vi "Tag FGV.vi"(0 "Operation":T4, 5 "Tag Name":string, 9 "Data":variant, 11 "error in (no error)":errorcluster, 12 "Tag Category":string) -> (2 "Alarm Array":T1[](array[typedef]), 3 "Process Name":string, 4 "Tag Names":string[](array[string]), 6 "Tag Values":dbl[](array[numeric]), 10 "Tag Value":dbl, 13 "Boolean alarm settings":T2, 14 "alarms":T3(array[cluster])=[{"alarm URL"="\\\\Nate-VM-LV2018\\sv_alarm_example\\my_number.Alarms.HiHi", "set time"=timestamp(3622821436.098553 s since 1904-01-01), "set user"="(Nobody)", "ack time"=timestamp(-9223372036854775808 s since 1904-01-01), "ack user"="", "clear time"=timestamp(-9223372036854775808 s since 1904-01-01), "clear user"="", "setpoint"=50.0, "value"=97.88238901880113, "priority"=1, "alarm area"="", "alarm description"="", "ack comment"="", "event?"=FALSE, "Refnum"=216172782113783811}] {"value" format="%.2f"; "setpoint" format="%.2f"; "clear time" format="%<%X\n%x>T"; "ack time" format="%<%X\n%x>T"; "set time" format="%<%X\n%x>T"}, 15 "error out":errorcluster)   [LabVIEW 2018, in "Dynamic Shared Variables.lvlib"]
doc: "Handles dynamic tag (shared variable) creation and release as well as alarm configuration and ack."
uses:
  Shared Variables/Dynamic Shared Variables.lvlib
  Tag FGV Operation Enum.ctl
  Numeric Alarm Settings Cluster.ctl
  Utilities/ISO 8601 type.ctl
  Shared Variables/URL Type Enum.ctl
  <vilib>/lvdsc/alarm/Acknowledge Alarms By Instance.vi
  <vilib>/lvdsc/variables/internal/Configure Alarming (Shared Variable, Numeric).vi
  <vilib>/lvdsc/variables/internal/Configure Alarming (Shared Variable, Boolean).vi
  <vilib>/lvdsc/variables/internal/Configure Alarming (Shared Variable, Enable Alarming).vi
  XML Config/XML Config.lvlib
  <vilib>/lvdsc/NI_DSC.lvlib
  <resource>/objmgr/nvio.rc
panel:
  out "Tag Category":string[](array[string])
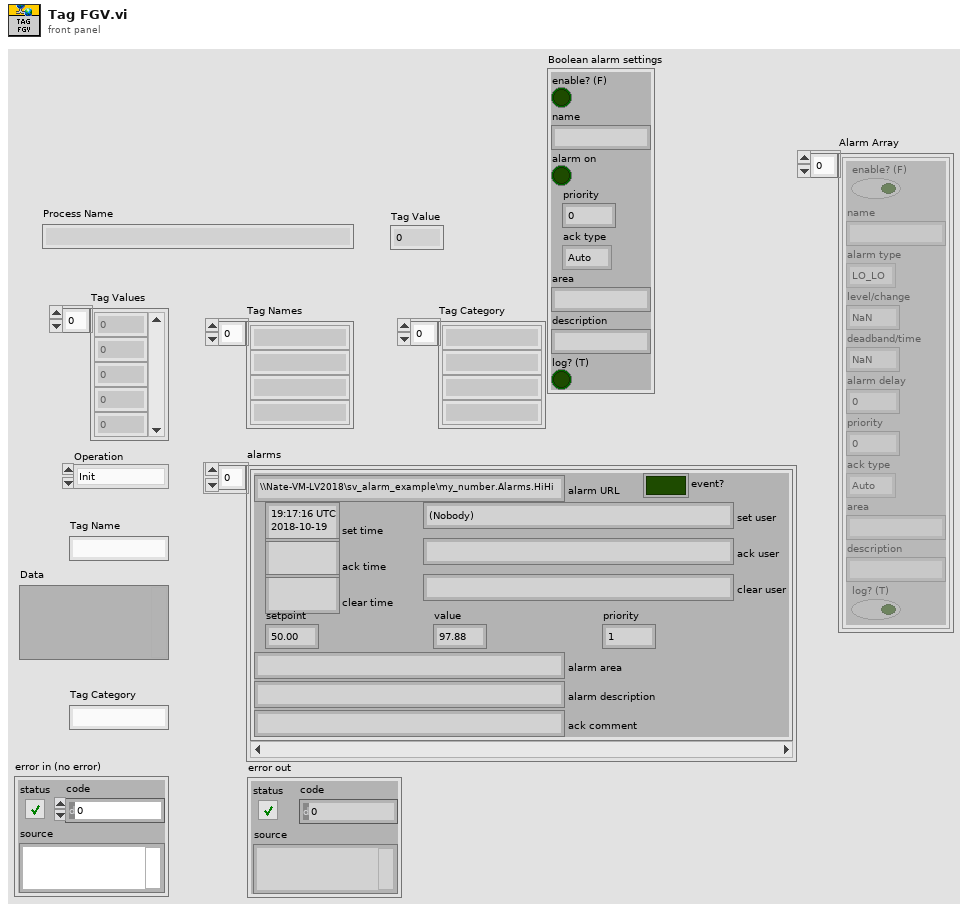
[diagram p1: front panel]
types:
  T1 = typedef "Numeric Alarm Settings Cluster.ctl" = cluster{"enable? (F)":bool, "name":string, "alarm type":enum16{"HI_HI", "HI", "LO", "LO_LO"}, "level/change":dbl, "deadband/time":dbl, "alarm delay":dbl, "priority":u32, "ack type":enum16{"Auto", "User", "None", "Each Occurrence"}, "area":string, "description":string, "log? (T)":bool}
  T2 = cluster{"enable? (F)":bool, "name":string, "alarm on":bool, "priority":u32, "ack type":enum16{"Auto", "User", "None", "Each Occurrence"}, "area":string, "description":string, "log? (T)":bool}
  T3 = cluster{"alarm URL":string, "set time":timestamp, "set user":string, "ack time":timestamp, "ack user":string, "clear time":timestamp, "clear user":string, "setpoint":dbl, "value":dbl, "priority":u32, "alarm area":string, "alarm description":string, "ack comment":string, "event?":bool, "Refnum":u64}[]
  T4 = typedef "Tag FGV Operation Enum.ctl" = enum16{"Init", "Set Notification Queue", "Create Tag", "Commit", "Write Tag (Numeric)", "Write Tag (Boolean)", "Read All Tags", "Read One Tag", "Delete Tag Category", "Set Alarm Parameters (Numeric)", "Set Alarm Parameters (Boolean)", "Enable All Alarms", "Disable All Alarms", "Delete All Tags", "Read Alarms", "Ack Alarm", "Read Alarm Parameters (Numeric)", "Read Alarm Parameters (Boolean)"}
  T5 = typedef "ISO 8601 type.ctl" = enum16{"full ISO 8601 UTC", "basic ISO8601 local", "Windows ISO 8601 UTC", "YYYY-MM-DD UTC", "full ISO 8601 local"}
  T6 = enum32{"u32BitField", "bool", "double", "string", "int8", "uint8", "int16", "uint16", "int32", "uint32", "int64", "uint64", "single", "double waveform", "int16 waveform", "array of boolean", "array of int8", "array of uint8", "array of int16", "array of uint16", "array of int32", "array of uint32", "array of int64", "array of uint64", "array of single", "array of double", "array of double waveform", "array of int16 waveform", "array of string", "variant", "timestamp", "fixed point", "custom"}
  T7 = typedef "Dynamic Shared Variables.lvlib/URL Type Enum.ctl" = enum16{"Tag", "HiHi", "Hi", "Lo", "LoLo", "Tag (Bool)"}
  T8 = cluster{"alarm URL":string, "set time":timestamp, "set user":string, "ack time":timestamp, "ack user":string, "clear time":timestamp, "clear user":string, "setpoint":dbl, "value":dbl, "priority":u32, "alarm area":string, "alarm description":string, "ack comment":string, "event?":bool, "Refnum":u64}
  T9 = enum16{"Auto", "User", "None", "Each Occurrence"}
  T10 = cluster{"enable? (F)":bool, "name":string, "alarm type":enum16{"HI_HI", "HI", "LO", "LO_LO"}, "level/change":dbl, "deadband/time":dbl, "priority":u32, "ack type":enum16{"Auto", "User", "None", "Each Occurrence"}, "area":string, "description":string, "log? (T)":bool}
  T11 = cluster{"enable? (F)":bool, "name":string, "alarm on":bool, "priority":u32, "ack type":enum16{"Auto", "User", "None", "Each Occurrence"}, "area":string, "description":string, "log? (T)":bool}[]
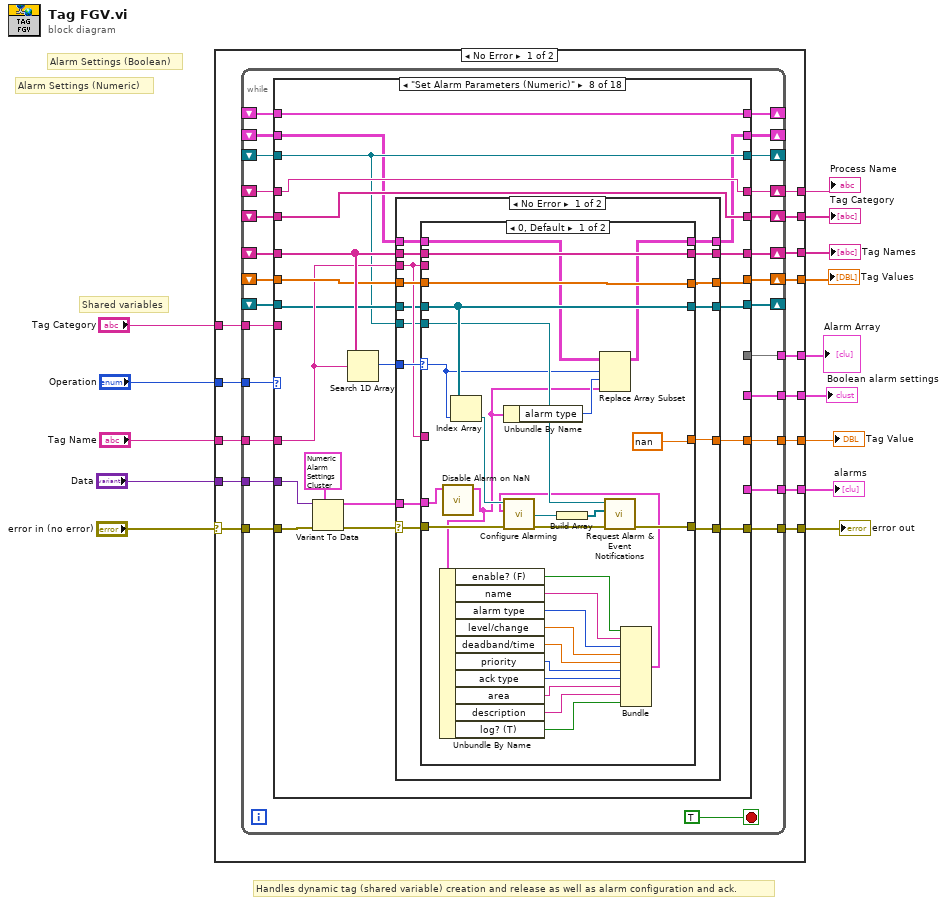
[diagram p0: block diagram]
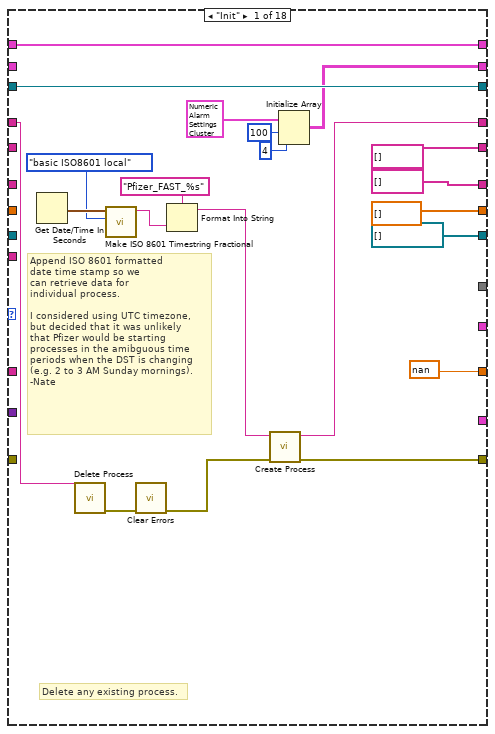
[diagram p2: hidden frame]
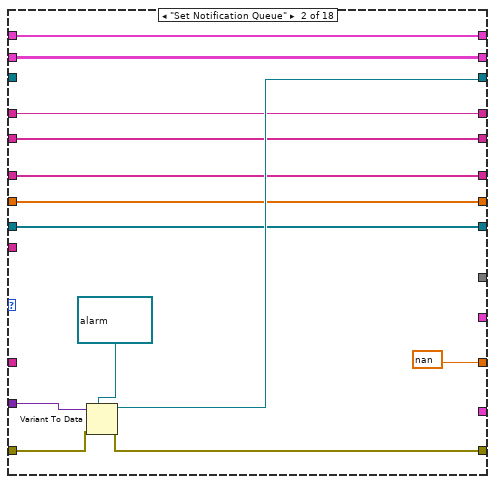
[diagram p3: hidden frame]
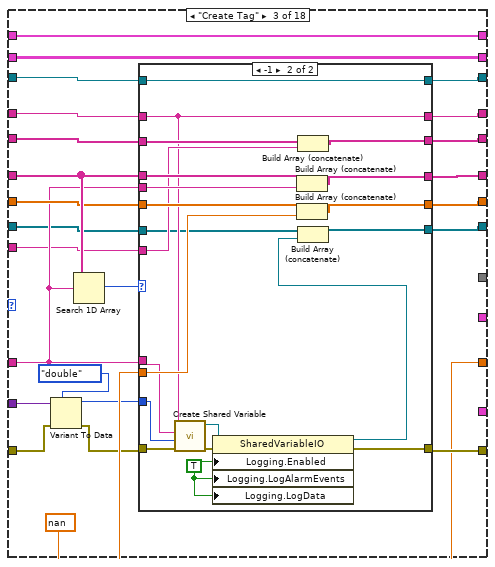
[diagram p4: hidden frame]
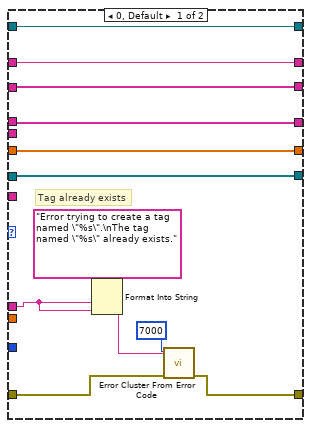
[diagram p5: hidden frame]
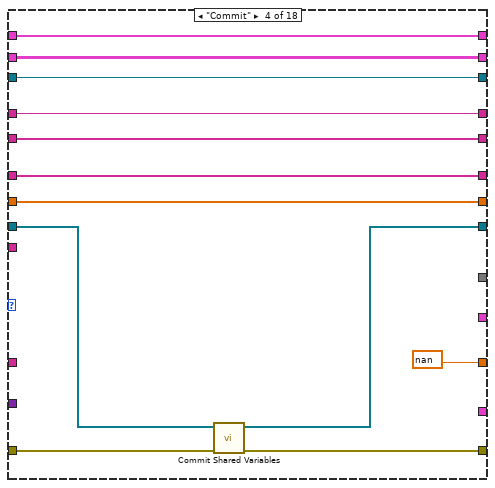
[diagram p6: hidden frame]
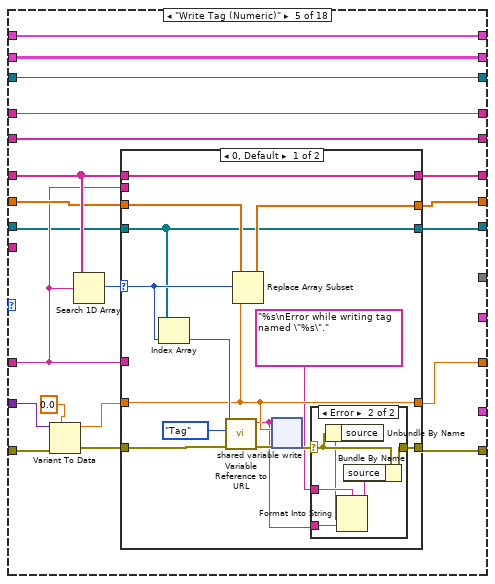
[diagram p7: hidden frame]
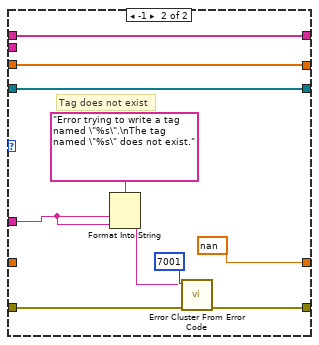
[diagram p9: hidden frame]
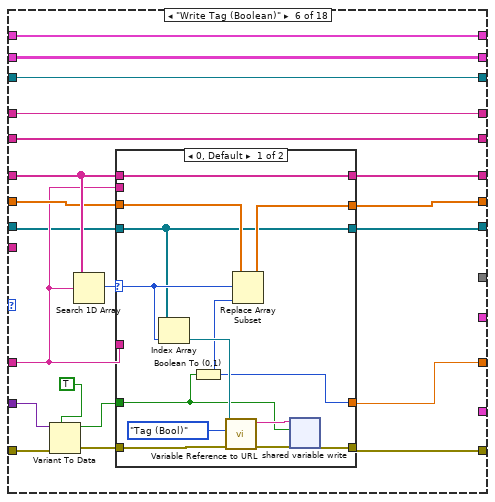
[diagram p10: hidden frame]
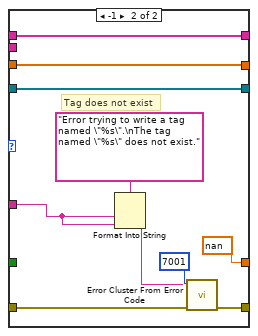
[diagram p11: hidden frame]
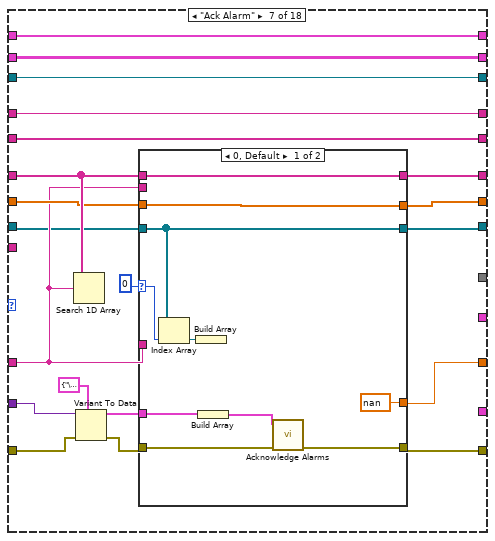
[diagram p12: hidden frame]
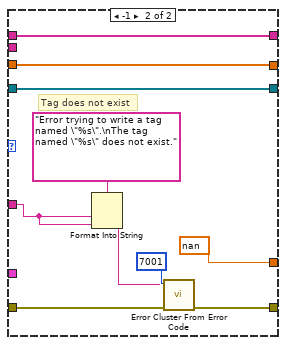
[diagram p13: hidden frame]
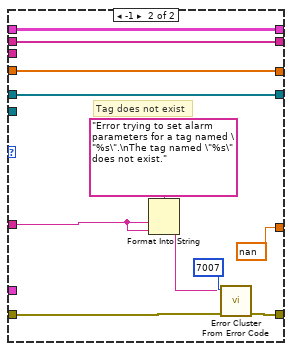
[diagram p14: hidden frame]
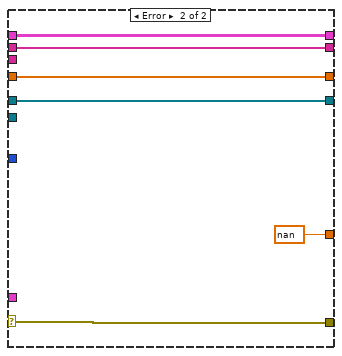
[diagram p15: hidden frame]
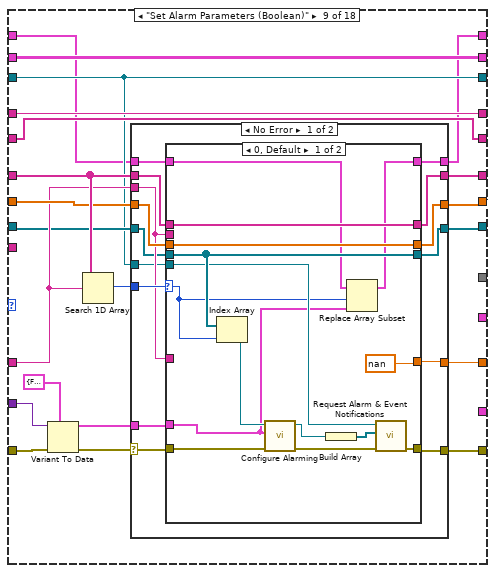
[diagram p16: hidden frame]
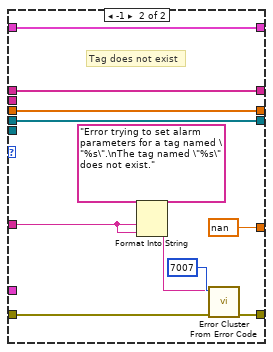
[diagram p17: hidden frame]
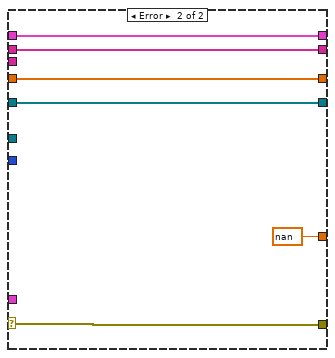
[diagram p18: hidden frame]
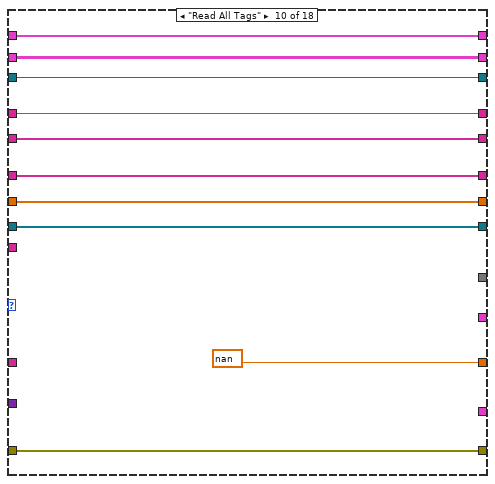
[diagram p19: hidden frame]
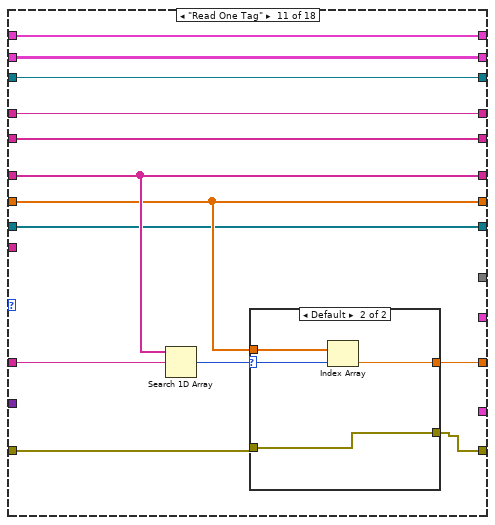
[diagram p20: hidden frame]
diagram:
  # "Alarm Settings (Boolean)"
  # "Alarm Settings (Numeric)"
  # "Handles dynamic tag (shared variable) creation and release as well as alarm configuration and ack."
  # "Shared variables"
  n1 = case shown="No Error" "error in (no error)" {
    selector: "error in (no error)" -> [w25 w618]
    tunnel: [w24 w618] -> w13
    tunnel: "Operation" -> [w28 _]
    tunnel: "Tag Name" -> [w27 _]
    tunnel: "Data" -> [w26 _]
    tunnel: [w23 _] -> w9
    tunnel: [w22 _] -> w8
    tunnel: [w21 nan ("Tag Value (NaN)")] -> w7
    tunnel: "Tag Category" -> [w20 _]
    tunnel: [w19 _] -> w5
    tunnel: [w18 _] -> w4
    tunnel: [w17 _] -> w3
    tunnel: [w16 _] -> w2
    tunnel: [w15 _] -> w1
    frame No Error {
      n2 = while {
        tunnel: w28 -> [w54]
        shift-right: [w52] -> w22
        shift-left: _ -> [w51]
        shift-right: [w53] -> w23
        shift-left: _ -> [w49]
        tunnel: w27 -> [w50]
        tunnel: w26 -> [w48]
        tunnel: w25 -> [w47]
        tunnel: [w45] -> w24
        tunnel: [w46] -> w21
        shift-right: [w44] -> w19
        shift-left: _ -> [w43]
        tunnel: w20 -> [w42]
        shift-right: [w41] -> w17
        shift-left: _ -> [w40]
        shift-right: [w39] -> _
        shift-left: _ -> [w38]
        tunnel: [w37] -> w18
        shift-right: [w36] -> _
        shift-left: _ -> [w35]
        shift-right: [w34] -> _
        shift-left: _ -> [w33]
        shift-right: [w32] -> _
        shift-left: _ -> [w31]
        tunnel: [w30] -> w16
        tunnel: [w29] -> w15
        stop <- TRUE stop-if-true
        n3 = case shown="\"Set Alarm Parameters (Numeric)\"" w54 {
          tunnel: [dbl[] [] ("Tag Values") w84 w109 w157 w174 w225 w269 w309 w390 w451 w462 w481 w497 w513 dbl[] [] ("Tag Values") w559 w576 w603] -> w53
          tunnel: [string[] [] ("Tag Names") w82 w111 w158 w176 w227 w271 w311 w392 w450 w464 w482 w498 w515 w543 w558 w572 w599] -> w52
          tunnel: w51 -> [_ w82 w112 w158 w177 w228 w272 w312 w393 w450 w464 w482 w498 w516 _ w558 w572 w599]
          tunnel: w50 -> [_ _ w108 _ w173 w224 w268 w308 w389 _ w463 _ _ w520 _ _ w567 w593]
          tunnel: w49 -> [_ w84 w110 w157 w175 w226 w270 w310 w391 w451 w462 w481 w497 w514 _ w559 w576 w603]
          tunnel: w48 -> [_ w88 w98 _ w162 w213 w261 w300 w381 _ _ _ _ _ _ _ _ _]
          tunnel: w47 -> [_ w86 w96 w150 w165 w216 w259 w298 w379 w449 w458 w477 w493 w510 w537 w563 w570 w597]
          tunnel: [w72 w85 w107 w156 w172 w223 w267 w307 w388 w449 w459 w475 w491 w508 w540 w562 w569 w596] -> w45
          tunnel: [nan ("Tag Value (NaN)") nan ("Tag Value (NaN)") w99 nan ("Tag Value (NaN)") w171 w222 w266 w306 w387 nan ("Tag Value (NaN)") w461 nan nan nan ("Tag Value (NaN)") nan ("Tag Value (NaN)") nan ("Tag Value (NaN)") nan ("Tag Value (NaN)") nan ("Tag Value (NaN)")] -> w46
          tunnel: [string[] [] ("Tag Names") w81 w104 w155 w170 w221 w265 w305 w386 w447 w457 w480 w496 w517 w543 w557 w577 w604] -> w44
          tunnel: w43 -> [_ w81 w106 w155 w170 w221 w265 w305 w386 w447 w457 w480 w496 w518 _ w557 w577 w604]
          tunnel: w42 -> [_ _ w105 _ _ _ _ _ _ _ _ _ _ w519 w546 _ _ _]
          tunnel: [w71 w80 w102 w154 w168 w219 w263 w303 w384 w445 w455 w479 w495 w507 w536 w556 w578 w605] -> w41
          tunnel: w40 -> [w62 w80 w103 w154 w168 w219 w263 w303 w384 w445 w455 w479 w495 w507 w536 w556 w578 w605]
          tunnel: [refnum<k21>[] [] w83 w101 w153 w167 w218 w262 w302 w383 w446 w456 w478 w494 w506 refnum<k21>[] [] w560 w575 w602] -> w39
          tunnel: w38 -> [_ w83 w100 w152 w169 w220 w264 w304 w385 w446 w456 w478 w494 w511 w544 w560 w575 w602]
          tunnel: [_ _ _ _ _ _ _ _ _ _ _ _ _ _ _ w564 _ _] -> w37
          tunnel: [w64 w87 w93 w151 w161 w212 w255 w297 w377 w444 w454 w473 w489 w505 w539 w555 w571 w598] -> w36
          tunnel: w35 -> [w64 _ w92 w151 w161 w212 w255 w297 w377 w444 w454 w473 w489 w505 w539 w555 w571 w598]
          tunnel: [w56 w78 w91 w148 w160 w211 w254 w296 w376 w443 w453 w472 w488 w504 w534 w554 w568 w606] -> w34
          tunnel: w33 -> [_ w78 w91 w148 w160 w211 w254 w295 w376 w443 w453 w472 w488 w504 w534 w554 w568 w606]
          tunnel: [w60 w77 w90 w147 w159 w210 w253 w294 w375 w442 w452 w471 w487 w503 w533 w553 w579 w595] -> w32
          tunnel: w31 -> [w60 w77 w90 w147 w159 w210 w253 w294 w374 w442 w452 w471 w487 w503 w533 w553 w579 w595]
          tunnel: [_ _ _ _ _ _ _ _ _ _ _ _ _ _ _ _ _ w594] -> w30
          tunnel: [_ _ _ _ _ _ _ _ _ _ _ _ _ _ _ _ w566 _] -> w29
          frame "Init" {
            # "Delete any existing process."
            # "Append ISO 8601 formatted\ndate time stamp so we\ncan retrieve data for\nindividual process.\n\nI considered using UTC timezone,\nbut decided that it was unlikely\nthat Pfizer would be starting\nprocesses in the amibguous time\nperiods when the DST is changing\n(e.g. 2 to 3 AM Sunday mornings).\n-Nate"
            n4 = Get Date/Time In Seconds() -> (seconds since 1Jan1904=w69:timestamp)
            n5 = call <vilib>:"Delete Process.vi"("process name"=w62) -> ("error out"=w63:errorcluster)  [unwired: 10 in]
            n6 = call "Make ISO 8601 Timestring Fractional.vi"("ISO 8601 type"=ISO_8601_type."basic ISO8601 local", "Time Stamp"=w69) -> ("ISO 8601 Timestring"=w66:string)  [unwired: 8 in, 1 out]
            n7 = call <vilib>:"Clear Errors.vi"("error in (no error)"=w63) -> ("error out"=w61:errorcluster)  [unwired: 5 in, 1 out]
            n8 = Format Into String(format string="Pfizer_FAST_%s", w66) -> (resulting string=w65:string)  [unwired: 2 in, 1 out]
            n9 = call "Create Process.vi"("error in (no error)"=w61, "process name"=w65) -> ("error out"=w72:errorcluster, "dup process name"=w71:string)  [unwired: 8 in]
            n10 = Initialize Array(T1 {"enable? (F)"=FALSE, "name"="", "alarm type"=enum."LO_LO", "level/change"=nan, "deadband/time"=nan, "alarm delay"=0.0, "priority"=0, "ack type"=enum."Auto", "area"="", "description"="", "log? (T)"=FALSE} ("numeric alarm settings out"), 100 ("dimension size"), 4 ("dimension size")) -> (w56:T1[][])
          }
          frame "Set Notification Queue" {
            n11 = Variant To Data(error in=w86, type=refnum<user-event> refnum ("notification refnum"), Variant=w88) -> (data=w87:refnum<user-event>, error out=w85:errorcluster)
          }
          frame "Create Tag" {
            w99 = nan ("Tag Value (NaN)")
            n12 = Variant To Data(error in=w96, type=T6."double" ("data type"), Variant=w98) -> (data=w94:T6, error out=w97:errorcluster)
            n13 = Search 1D Array(1D array=w112, element=w108) -> (index of element=w113:i32)  [unwired: 1 in]
            n14 = case shown="-1" w113 {
              tunnel: w108 -> [_ w146]
              tunnel: w112 -> [w125 w145]
              tunnel: [w125 w144] -> w111
              tunnel: w110 -> [w124 w143]
              tunnel: w99 -> [_ w142]
              tunnel: [w124 w141] -> w109
              tunnel: w97 -> [w123 w136]
              tunnel: w108 -> [w120 w137]
              tunnel: [w118 w126] -> w107
              tunnel: w106 -> [w117 w140]
              tunnel: w105 -> [_ w139]
              tunnel: [w117 w138] -> w104
              tunnel: w103 -> [w116 w135]
              tunnel: [w116 w135] -> w102
              tunnel: [w115 w134] -> w101
              tunnel: w100 -> [w115 w133]
              tunnel: w94 -> [_ w129]
              tunnel: [w114 w127] -> w93
              tunnel: w92 -> [w114 w127]
              frame 0, Default {
                # "Tag already exists"
                n15 = Format Into String(format string="Error trying to create a tag named \"%s\".\nThe tag named \"%s\" already exists.", w120, w120) -> (resulting string=w119:string)  [unwired: 2 in, 1 out]
                n16 = call <vilib>:"Error Cluster From Error Code.vi"("error in (no error)"=w123, "error message (\"\")"=w119, "error code (0)"=7000) -> ("error out"=w118:errorcluster)  [unwired: 6 in]
              }
              frame -1 {
                w130 = TRUE ("Logging.LogAlarmEvents")
                n17 = call "Create Shared Variable.vi"("error in (no error)"=w136, "data type"=w129, "shared variable name"=w137, "process name out"=w135) -> ("error out"=w132:errorcluster, "shared variable"=w128:refnum<k21>)  [unwired: 6 in]
                n18 = property class="SharedVariableIO"(reference=w128, error in=w132, "Logging.Enabled"=w130, "Logging.LogAlarmEvents"=w130, "Logging.LogData"=w130) -> (reference out=w131:refnum<k21>, error out=w126:errorcluster)
                n19 = Build Array (concatenate)(w145, w146) -> (w144:string[])
                n20 = Build Array (concatenate)(w143, w142) -> (w141:dbl[])
                n21 = Build Array (concatenate)(w140, w139) -> (w138:string[])
                n22 = Build Array (concatenate)(w133, w131) -> (w134:refnum<k21>[])
              }
            }
          }
          frame "Commit" {
            n23 = call <vilib>:"Commit Shared Variables.vi"("error in (no error)"=w150, "shared variables"=w152) -> ("error out"=w156:errorcluster, "shared variables out"=w153:refnum<k21>[])  [unwired: 8 in]
          }
          frame "Write Tag (Numeric)" {
            n24 = Variant To Data(error in=w165, type=0.0, Variant=w162) -> (data=w163:dbl, error out=w164:errorcluster)
            n25 = Search 1D Array(1D array=w177, element=w173) -> (index of element=w178:i32)  [unwired: 1 in]
            n26 = case shown="0, Default" w178 {
              selector: w178 -> [w189 _]
              tunnel: w173 -> [_ _]
              tunnel: w177 -> [w192 w209]
              tunnel: [w192 w209] -> w176
              tunnel: w175 -> [w191 w208]
              tunnel: w163 -> [w186 _]
              tunnel: [w190 w208] -> w174
              tunnel: w164 -> [w185 w207]
              tunnel: w173 -> [_ w204]
              tunnel: [w181 w202] -> w172
              tunnel: [w186 nan ("Tag Value (NaN)")] -> w171
              tunnel: w169 -> [w183 w200]
              tunnel: [w183 w200] -> w167
              frame 0, Default {
                n27 = Index Array(array=w183, index=w189) -> (element=w188:refnum<k21>)
                n28 = call "Variable Reference to URL.vi"("error in (no error)"=w185, "URL type"=URL_Type_Enum."Tag", "variable reference"=w188) -> ("error out"=w184:errorcluster, "URL"=w179:string)  [unwired: 7 in]
                n29 = Replace Array Subset(array=w191, new element=w186, index=w189) -> (w190:dbl[])
                n30 = shared-variable-write(w179, w184, w186) -> (w182:errorcluster)  [unwired: 1 out]
                n31 = case shown="Error" w182 {
                  selector: w182 -> [w193 w199]
                  tunnel: [w193 w198] -> w181
                  tunnel: "%s\nError while writing tag named \"%s\"." ("format string") -> [_ w197]
                  tunnel: w179 -> [_ w194]
                  frame No Error {
                  }
                  frame Error {
                    n32 = Unbundle By Name(w199) -> ("source"=w196:string)
                    n33 = Format Into String(format string=w197, w196, w194) -> (resulting string=w195:string)  [unwired: 2 in, 1 out]
                    n34 = Bundle By Name(cluster=w199, "source"=w195) -> (w198:errorcluster)
                  }
                }
              }
              frame -1 {
                # "Tag does not exist"
                n35 = Format Into String(format string="Error trying to write a tag named \"%s\".\nThe tag named \"%s\" does not exist.", w204, w204) -> (resulting string=w203:string)  [unwired: 2 in, 1 out]
                n36 = call <vilib>:"Error Cluster From Error Code.vi"("error in (no error)"=w207, "error message (\"\")"=w203, "error code (0)"=7001) -> ("error out"=w202:errorcluster)  [unwired: 6 in]
              }
            }
          }
          frame "Write Tag (Boolean)" {
            n37 = Variant To Data(error in=w216, type=TRUE, Variant=w213) -> (data=w214:bool, error out=w215:errorcluster)
            n38 = Search 1D Array(1D array=w228, element=w224) -> (index of element=w229:i32)  [unwired: 1 in]
            n39 = case shown="0, Default" w229 {
              selector: w229 -> [w239 _]
              tunnel: w224 -> [_ _]
              tunnel: w228 -> [w242 w252]
              tunnel: [w242 w252] -> w227
              tunnel: w226 -> [w241 w251]
              tunnel: w214 -> [w231 _]
              tunnel: [w240 w251] -> w225
              tunnel: w215 -> [w235 w250]
              tunnel: w224 -> [_ w247]
              tunnel: [w233 w245] -> w223
              tunnel: [w230 nan ("Tag Value (NaN)")] -> w222
              tunnel: w220 -> [w232 w243]
              tunnel: [w232 w243] -> w218
              frame 0, Default {
                n40 = Index Array(array=w232, index=w239) -> (element=w238:refnum<k21>)
                n41 = Boolean To (0,1)(Boolean=w231) -> (0, 1=w230:i16)
                n42 = call "Variable Reference to URL.vi"("error in (no error)"=w235, "URL type"=URL_Type_Enum."Tag (Bool)", "variable reference"=w238) -> ("error out"=w234:errorcluster, "URL"=w236:string)  [unwired: 7 in]
                n43 = Replace Array Subset(array=w241, new element=w230, index=w239) -> (w240:dbl[])
                n44 = shared-variable-write(w236, w234, w231) -> (w233:errorcluster)  [unwired: 1 out]
              }
              frame -1 {
                # "Tag does not exist"
                n45 = Format Into String(format string="Error trying to write a tag named \"%s\".\nThe tag named \"%s\" does not exist.", w247, w247) -> (resulting string=w246:string)  [unwired: 2 in, 1 out]
                n46 = call <vilib>:"Error Cluster From Error Code.vi"("error in (no error)"=w250, "error message (\"\")"=w246, "error code (0)"=7001) -> ("error out"=w245:errorcluster)  [unwired: 6 in]
              }
            }
          }
          frame "Ack Alarm" {
            n47 = Search 1D Array(1D array=w272, element=w268) -> ()  [unwired: 1 in, 1 out]
            n48 = Variant To Data(error in=w259, type=T8 {"alarm URL"="\\\\Nate-VM-LV2018\\Pfizer FAST\\TT1.Alarms.TT1:LoLo", "set time"=timestamp(3634824876.5239263 s since 1904-01-01), "set user"="(Nobody)", "ack time"=timestamp(-9223372036854775808 s since 1904-01-01), "ack user"="", "clear time"=timestamp(-9223372036854775808 s since 1904-01-01), "clear user"="", "setpoint"=20.0, "value"=19.923748781652513, "priority"=100, "alarm area"="", "alarm description"="", "ack comment"="", "event?"=FALSE, "Refnum"=216172782113783885} ("Alarm"), Variant=w261) -> (data=w258:T8, error out=w260:errorcluster)
            n49 = case shown="0, Default" 0 ("index of element") {
              selector: 0 ("index of element") -> [w281 _]
              tunnel: w268 -> [_ _]
              tunnel: w272 -> [w282 w292]
              tunnel: [w282 w292] -> w271
              tunnel: w270 -> [w278 w291]
              tunnel: [w278 w291] -> w269
              tunnel: w260 -> [w276 w290]
              tunnel: w268 -> [_ w287]
              tunnel: [w275 w285] -> w267
              tunnel: [nan ("Tag Value (NaN)") nan ("Tag Value (NaN)")] -> w266
              tunnel: w264 -> [w280 w283]
              tunnel: [w280 w283] -> w262
              tunnel: w258 -> [w274 _]
              frame 0, Default {
                n50 = Index Array(array=w280, index=w281) -> (element=w279:refnum<k21>)
                n51 = Build Array(w279) -> ()  [unwired: 1 out]
                n52 = Build Array(w274) -> (w273:T3)
                n53 = call-poly <vilib>:"Acknowledge Alarms.vi"("error in (no error)"=w276, "alarms"=w273) -> ("error out"=w275:errorcluster)  [unwired: 9 in]
              }
              frame -1 {
                # "Tag does not exist"
                n54 = Format Into String(format string="Error trying to write a tag named \"%s\".\nThe tag named \"%s\" does not exist.", w287, w287) -> (resulting string=w286:string)  [unwired: 2 in, 1 out]
                n55 = call <vilib>:"Error Cluster From Error Code.vi"("error in (no error)"=w290, "error message (\"\")"=w286, "error code (0)"=7001) -> ("error out"=w285:errorcluster)  [unwired: 6 in]
              }
            }
          }
          frame "Set Alarm Parameters (Numeric)" {
            n56 = Variant To Data(error in=w298, type=T1 {"enable? (F)"=FALSE, "name"="", "alarm type"=enum."LO_LO", "level/change"=nan, "deadband/time"=nan, "alarm delay"=0.0, "priority"=0, "ack type"=enum."Auto", "area"="", "description"="", "log? (T)"=FALSE} ("numeric alarm settings out"), Variant=w300) -> (data=w301:T1, error out=w299:errorcluster)
            n57 = Search 1D Array(1D array=w312, element=w308) -> (index of element=w313:i32)  [unwired: 1 in]
            n58 = case shown="No Error" w299 {
              selector: w299 -> [w317 w369]
              tunnel: w313 -> [w328 _]
              tunnel: w312 -> [w327 w371]
              tunnel: [w326 w371] -> w311
              tunnel: w310 -> [w325 w372]
              tunnel: w301 -> [w324 _]
              tunnel: [w323 w372] -> w309
              tunnel: w308 -> [w322 _]
              tunnel: [w321 w369] -> w307
              tunnel: [w320 nan ("Tag Value (NaN)")] -> w306
              tunnel: w304 -> [w319 w373]
              tunnel: [w318 w373] -> w302
              tunnel: w297 -> [w316 _]
              tunnel: [w315 w368] -> w296
              tunnel: w295 -> [w314 w368]
              frame No Error {
                n59 = case shown="0, Default" w328 {
                  selector: w328 -> [w344 _]
                  tunnel: w322 -> [_ _]
                  tunnel: w327 -> [w356 w367]
                  tunnel: [w356 w367] -> w326
                  tunnel: w325 -> [w351 w366]
                  tunnel: w324 -> [w350 _]
                  tunnel: [w351 w366] -> w323
                  tunnel: w317 -> [w353 w365]
                  tunnel: w322 -> [_ w358]
                  tunnel: [w345 w361] -> w321
                  tunnel: [nan nan ("Tag Value (NaN)")] -> w320
                  tunnel: w319 -> [w355 w359]
                  tunnel: [w355 w359] -> w318
                  tunnel: w316 -> [w347 _]
                  tunnel: [w343 w357] -> w315
                  tunnel: w314 -> [w342 w357]
                  frame 0, Default {
                    n60 = call "Disable Alarm on NaN.vi"("numeric alarm settings in"=w350) -> ("numeric alarm settings out"=w340:T1)  [unwired: 10 in]
                    n61 = Unbundle By Name(w340) -> ("enable? (F)"=w339:bool, "name"=w338:string, "alarm type"=w337:enum16{"HI_HI", "HI", "LO", "LO_LO"}, "level/change"=w336:dbl, "deadband/time"=w335:dbl, "priority"=w334:u32, "ack type"=w333:T9, "area"=w332:string, "description"=w331:string, "log? (T)"=w330:bool)
                    n62 = Index Array(array=w355, index=w344) -> (element=w354:refnum<k21>)
                    n63 = Unbundle By Name(w340) -> ("alarm type"=w341:enum16{"HI_HI", "HI", "LO", "LO_LO"})
                    n64 = Replace Array Subset(array=w342, new element=w340, index (row)=w344, index (col)=w341) -> (w343:T1[][])
                    n65 = Bundle("enable? (F)"=w339, "name"=w338, "alarm type"=w337, "level/change"=w336, "deadband/time"=w335, "priority"=w334, "ack type"=w333, "area"=w332, "description"=w331, "log? (T)"=w330) -> (w329:T10)  [unwired: 1 in]
                    n66 = call-poly <vilib>:"Configure Alarming.vi"("error in (no error)"=w353, "numeric alarm settings"=w329, "variable reference in"=w354) -> ("error out"=w346:errorcluster, "variable reference out"=w348:refnum<k21>)  [unwired: 7 in]
                    n67 = Build Array(w348) -> (w349:refnum<k21>[])
                    n68 = call <vilib>:"Request Alarm & Event Notifications.vi"("error in (no error)"=w346, "shared variables"=w349, "notification refnum"=w347) -> ("error out"=w345:errorcluster)  [unwired: 6 in, 2 out]
                  }
                  frame -1 {
                    # "Tag does not exist"
                    n69 = Format Into String(format string="Error trying to set alarm parameters for a tag named \"%s\".\nThe tag named \"%s\" does not exist.", w358, w358) -> (resulting string=w362:string)  [unwired: 2 in, 1 out]
                    n70 = call <vilib>:"Error Cluster From Error Code.vi"("error in (no error)"=w365, "error message (\"\")"=w362, "error code (0)"=7007) -> ("error out"=w361:errorcluster)  [unwired: 6 in]
                  }
                }
              }
              frame Error {
              }
            }
          }
          frame "Set Alarm Parameters (Boolean)" {
            n71 = Variant To Data(error in=w379, type=T2 {"enable? (F)"=FALSE, "name"="Boolean", "alarm on"=TRUE, "priority"=1, "ack type"=enum."Auto", "area"="", "description"="", "log? (T)"=TRUE} ("Boolean alarm settings"), Variant=w381) -> (data=w382:T2, error out=w380:errorcluster)
            n72 = Search 1D Array(1D array=w393, element=w389) -> (index of element=w394:i32)  [unwired: 1 in]
            n73 = case shown="No Error" w380 {
              selector: w380 -> [w398 w437]
              tunnel: w394 -> [w409 _]
              tunnel: w393 -> [w408 w439]
              tunnel: [w407 w439] -> w392
              tunnel: w391 -> [w406 w440]
              tunnel: w382 -> [w405 _]
              tunnel: [w404 w440] -> w390
              tunnel: w389 -> [w403 _]
              tunnel: [w402 w437] -> w388
              tunnel: [w401 nan ("Tag Value (NaN)")] -> w387
              tunnel: w385 -> [w400 w441]
              tunnel: [w399 w441] -> w383
              tunnel: w377 -> [w397 _]
              tunnel: [w396 w436] -> w375
              tunnel: w374 -> [w395 w436]
              frame No Error {
                n74 = case shown="0, Default" w409 {
                  selector: w409 -> [w413 _]
                  tunnel: w403 -> [_ _]
                  tunnel: w408 -> [w424 w435]
                  tunnel: [w424 w435] -> w407
                  tunnel: w406 -> [w419 w434]
                  tunnel: w405 -> [w411 _]
                  tunnel: [w419 w434] -> w404
                  tunnel: w398 -> [w421 w433]
                  tunnel: w403 -> [_ w426]
                  tunnel: [w414 w429] -> w402
                  tunnel: [nan nan ("Tag Value (NaN)")] -> w401
                  tunnel: w400 -> [w423 w427]
                  tunnel: [w423 w427] -> w399
                  tunnel: w397 -> [w417 _]
                  tunnel: [w412 w425] -> w396
                  tunnel: w395 -> [w410 w425]
                  frame 0, Default {
                    n75 = Index Array(array=w423, index=w413) -> (element=w422:refnum<k21>)
                    n76 = call-poly <vilib>:"Configure Alarming.vi"("error in (no error)"=w421, "Boolean alarm settings"=w411, "variable reference in"=w422) -> ("error out"=w415:errorcluster, "variable reference out"=w416:refnum<k21>)  [unwired: 7 in]
                    n77 = Build Array(w416) -> (w418:refnum<k21>[])
                    n78 = Replace Array Subset(array=w410, new element=w411, index=w413) -> (w412:T11)
                    n79 = call <vilib>:"Request Alarm & Event Notifications.vi"("error in (no error)"=w415, "shared variables"=w418, "notification refnum"=w417) -> ("error out"=w414:errorcluster)  [unwired: 6 in, 2 out]
                  }
                  frame -1 {
                    # "Tag does not exist"
                    n80 = Format Into String(format string="Error trying to set alarm parameters for a tag named \"%s\".\nThe tag named \"%s\" does not exist.", w426, w426) -> (resulting string=w430:string)  [unwired: 2 in, 1 out]
                    n81 = call <vilib>:"Error Cluster From Error Code.vi"("error in (no error)"=w433, "error message (\"\")"=w430, "error code (0)"=7007) -> ("error out"=w429:errorcluster)  [unwired: 6 in]
                  }
                }
              }
              frame Error {
              }
            }
          }
          frame "Read All Tags" {
          }
          frame "Read One Tag" {
            n82 = Search 1D Array(1D array=w464, element=w463) -> (index of element=w460:i32)  [unwired: 1 in]
            n83 = case shown="Default" w460 {
              selector: w460 -> [_ w468]
              tunnel: w462 -> [_ w470]
              tunnel: [nan ("Tag Value (NaN)") w469] -> w461
              tunnel: [errorcluster {"status"=TRUE, "code"=7002, "source"="Tag Name not found in Tag Names in Tag FGV.vi"} ("error IO") w467] -> w459
              tunnel: w458 -> [_ w467]
              frame -1 {
              }
              frame Default {
                n84 = Index Array(array=w470, index=w468) -> (element=w469:dbl)
              }
            }
          }
          frame "Enable All Alarms" {
            n85 = for {
              tunnel: w478 -> [w485] mode=indexing
              tunnel: w477 -> [w484]
              tunnel: [w483] -> w476 mode=indexing
              n86 = call-poly <vilib>:"Configure Alarming.vi"("error in (no error)"=w484, "enable? (F)"=TRUE, "variable reference in"=w485) -> ("error out"=w483:errorcluster)  [unwired: 7 in, 1 out]
            }
            n87 = Merge Errors(w476) -> (w475:errorcluster)
          }
          frame "Disable All Alarms" {
            n88 = for {
              tunnel: w494 -> [w501] mode=indexing
              tunnel: w493 -> [w500]
              tunnel: [w499] -> w492 mode=indexing
              n89 = call-poly <vilib>:"Configure Alarming.vi"("error in (no error)"=w500, "enable? (F)"=FALSE, "variable reference in"=w501) -> ("error out"=w499:errorcluster)  [unwired: 7 in, 1 out]
            }
            n90 = Merge Errors(w492) -> (w491:errorcluster)
          }
          frame "Delete Tag Category" {
            # "Delete all tags matching the tag category. This is to support when\na user picks a new DAQmx task, and the channels (i.e. tags) of the\nnew task will replace all the channels (i.e. tags) of the old task.\n\nThus this case is used to delete all the DAQ tags."
            n91 = for {
              tunnel: w520 -> [_]
              tunnel: w518 -> [w527] mode=indexing
              tunnel: w516 -> [w526] mode=indexing
              tunnel: w514 -> [w525] mode=indexing
              tunnel: w519 -> [w528]
              tunnel: [w527] -> w517 mode=indexing if=w521
              tunnel: [w526] -> w515 mode=indexing if=w521
              tunnel: [w525] -> w513 mode=indexing if=w521
              tunnel: w511 -> [w522] mode=indexing
              tunnel: w510 -> [w524]
              tunnel: [w523] -> w509 mode=indexing
              tunnel: [w522] -> w506 mode=indexing if=w521
              n92 = Not Equal?(x=w527, y=w528) -> (x != y?=w521:bool)
              n93 = case shown="False" w521 {
                tunnel: w522 -> [w531 _]
                tunnel: w524 -> [w530 w532]
                tunnel: [w529 w532] -> w523
                frame False {
                  n94 = call <vilib>:"Delete Shared Variable.vi"("error in (no error)"=w530, "shared variable"=w531) -> ("error out"=w529:errorcluster)  [unwired: 9 in]
                }
                frame True {
                }
              }
            }
            n95 = Merge Errors(w509) -> (w508:errorcluster)
          }
          frame "Delete All Tags" {
            w543 = string[] [] ("Tag Names")
            # "Delete all tags matching the tag category. This is to support when\na user picks a new DAQmx task, and the channels (i.e. tags) of the\nnew task will replace all the channels (i.e. tags) of the old task.\n\nThus this case is used to delete all the DAQ tags."
            n96 = call <vilib>:"Disable Alarm & Event Notifications.vi"("error in (no error)"=w537, "notification refnum"=w539) -> ("error out"=w538:errorcluster)  [unwired: 9 in]
            n97 = for {
              tunnel: w546 -> [_]
              tunnel: w544 -> [w550] mode=indexing
              tunnel: w538 -> [w552]
              tunnel: [w551] -> w535 mode=indexing
              n98 = call <vilib>:"Delete Shared Variable.vi"("error in (no error)"=w552, "shared variable"=w550) -> ("error out"=w551:errorcluster)  [unwired: 9 in]
            }
            n99 = flat-sequence {
              tunnel: [w548] -> w540
              tunnel: w536 -> [w547]
              tunnel: w535 -> [_]
              frame #0 {
                n100 = call <vilib>:"Delete Process.vi"("process name"=w547) -> ("error out"=w549:errorcluster)  [unwired: 10 in]
                n101 = call <vilib>:"Clear Errors.vi"("error in (no error)"=w549) -> ("error out"=w548:errorcluster)  [unwired: 5 in, 1 out]
              }
            }
          }
          frame "Read Alarms" {
            n102 = call <vilib>:"Read Alarms.vi"("error in (no error)"=w563, "timeout (s)"=1, "shared variables"=w560) -> ("error out"=w562:errorcluster, "alarms"=w564:T3)  [unwired: 7 in]
          }
          frame "Read Alarm Parameters (Numeric)" {
            n103 = Search 1D Array(1D array=w572, element=w567) -> (index of element=w573:i32)  [unwired: 1 in]
            n104 = case shown="0, Default" w573 {
              selector: w573 -> [w581 _]
              tunnel: [w586 w589] -> w569
              tunnel: w570 -> [w586 _]
              tunnel: w568 -> [w585 _]
              tunnel: [w580 T1[] [{"enable? (F)"=FALSE, "name"="", "alarm type"=enum."LO_LO", "level/change"=nan, "deadband/time"=nan, "alarm delay"=0.0, "priority"=0, "ack type"=enum."Auto", "area"="", "description"="", "log? (T)"=FALSE}]] -> w566
              tunnel: w567 -> [_ w588]
              frame 0, Default {
                n105 = Index Array(array=w585, index (row)=w581) -> (element=w584:T1[])  [unwired: 1 in]
                n106 = Array Subset(array=w584, index=0, length=4) -> (w580:T1[])
              }
              frame -1 {
                (unwired) nan ("Tag Value (NaN)")
                # "Tag does not exist"
                n107 = Format Into String(format string="Error trying to retrieve alarm parameters for a tag named \"%s\".\nThe tag named \"%s\" does not exist.", w588, w588) -> (resulting string=w590:string)  [unwired: 2 in, 1 out]
                n108 = call <vilib>:"Error Cluster From Error Code.vi"("error message (\"\")"=w590, "error code (0)"=7007) -> ("error out"=w589:errorcluster)  [unwired: 7 in]
              }
            }
          }
          frame "Read Alarm Parameters (Boolean)" {
            n109 = Search 1D Array(1D array=w599, element=w593) -> (index of element=w600:i32)  [unwired: 1 in]
            n110 = case shown="-1" w600 {
              selector: w600 -> [w608 _]
              tunnel: [w610 w613] -> w596
              tunnel: w597 -> [w610 _]
              tunnel: w595 -> [w609 _]
              tunnel: [w607 T2 {"enable? (F)"=FALSE, "name"="", "alarm on"=FALSE, "priority"=0, "ack type"=enum."Auto", "area"="", "description"="", "log? (T)"=FALSE} ("Boolean alarm settings")] -> w594
              tunnel: w593 -> [_ w611]
              frame 0, Default {
                n111 = Index Array(array=w609, index=w608) -> (element=w607:T2)
              }
              frame -1 {
                (unwired) nan ("Tag Value (NaN)")
                # "Tag does not exist"
                n112 = Format Into String(format string="Error trying to retrieve alarm parameters for a tag named \"%s\".\nThe tag named \"%s\" does not exist.", w611, w611) -> (resulting string=w614:string)  [unwired: 2 in, 1 out]
                n113 = call <vilib>:"Error Cluster From Error Code.vi"("error message (\"\")"=w614, "error code (0)"=7007) -> ("error out"=w613:errorcluster)  [unwired: 7 in]
              }
            }
          }
        }
      }
    }
    frame Error {
    }
  }
  "error out" <- w13
  "Tag Names" <- w8
  "Tag Values" <- w9
  "Tag Value" <- w7
  "Tag Category" <- w5
  "alarms" <- w4
  "Process Name" <- w3
  "Boolean alarm settings" <- w2
  "Alarm Array" <- w1
